vi "ActionVIOnSave.vi"(8 "error in (no error)":errorcluster, 11 "Device Item Ref in":T1 format="%.0x") -> (0 "error out":errorcluster, 3 "Device Item Ref out":T1 format="%.0x")   [LabVIEW 2016]
uses:
  <vilib>/NI Veristand/Custom Device API/Custom Device Item Ref.ctl
  UDP-Custom-Device System Explorer.lvlib
  <vilib>/NI VeriStand/Custom Device API/Custom Device API.lvlib
  Shared/Constants.vi
  Shared/UDP-Custom-Device Shared.lvlib
  <vilib>/NI VeriStand/Custom Device Tools/Custom Device Utility Library/Custom Device Utility Library.lvlib
  <vilib>/NI Veristand/Custom Device API/Get Item Property (Boolean).vi
  <vilib>/NI Veristand/Custom Device API/Get Item Property (Path).vi
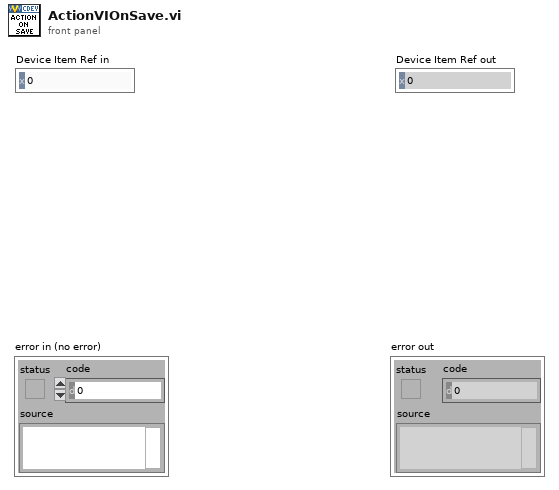
[diagram p1: front panel]
types:
  T1 = typedef "Custom Device API.lvlib/Custom Device Item Ref.ctl" = u64
  T2 = typedef "UDP-Custom-Device System Explorer.lvlib/XML - Header Data.ctl" = cluster{"Revision (\"Major.Minor.Fix.Build\")":string, "Creation Date (\"yyyy-mm-dd\")":string, "Controller Name":string}
  T3 = typedef "UDP-Custom-Device System Explorer.lvlib/XML - Group.ctl" = cluster{"Freq":i32, "Tx Channels":T4[], "Rx Channels":T4[]}
  T4 = typedef "UDP-Custom-Device System Explorer.lvlib/XML - Channel.ctl" = cluster{"Channel Name":string, "Data Type":u16, "Description":string, "Unit":string}
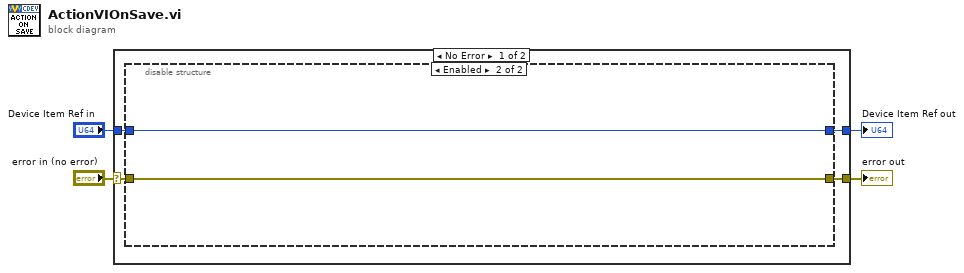
[diagram p0: block diagram]
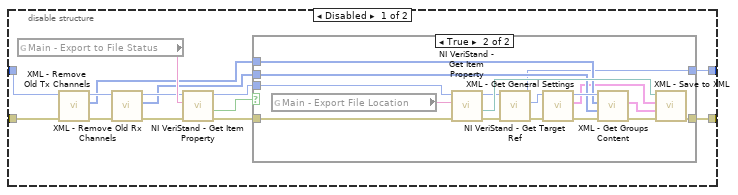
[diagram p2: hidden frame]
diagram:
  n1 = case shown="No Error" "error in (no error)" {
    selector: "error in (no error)" -> [w7 w45]
    tunnel: [w6 w45] -> w3
    tunnel: "Device Item Ref in" -> [w8 w44]
    tunnel: [w5 w44] -> w1
    frame No Error {
      n2 = disable-structure shown="Enabled" {
        disable-tunnel: w8 -> [w22 w43]
        disable-tunnel: w7 -> [w21 w42]
        disable-tunnel: [w10 w42] -> w6
        disable-tunnel: [w9 w43] -> w5
        frame Disabled {
          n3 = global read "Constants.vi" "Main - Export to File Status"() -> (w18:string)
          n4 = call "XML - Remove Old Tx Channels.vi"("error in (no error)"=w21, "Device Item Ref in"=w22) -> ("error out"=w20:errorcluster, "Tx Dependent Refs"=w12:T1[], "Device Item Ref out"=w19:T1)  [unwired: 7 in]
          n5 = call "XML - Remove Old Rx Channels.vi"("error in (no error)"=w20, "Device Item Ref in"=w19) -> ("error out"=w16:errorcluster, "Rx Dependent Refs"=w11:T1[], "Device Item Ref out"=w17:T1)  [unwired: 7 in]
          n6 = call-poly <vilib>:"NI VeriStand - Get Item Property.vi"("error in (no error)"=w16, "Property Name"=w18, "Item Ref in"=w17) -> ("error out"=w14:errorcluster, "Value"=w15:bool, "Item Ref out"=w13:T1)  [unwired: 5 in, 1 out]
          n7 = case shown="True" w15 {
            tunnel: w14 -> [w24 w41]
            tunnel: w13 -> [w23 w40]
            tunnel: w12 -> [_ w32]
            tunnel: w11 -> [_ w31]
            tunnel: [w24 w26] -> w10
            tunnel: [w23 w25] -> w9
            frame False {
            }
            frame True {
              n8 = global read "Constants.vi" "Main - Export File Location"() -> (w39:string)
              n9 = call-poly <vilib>:"NI VeriStand - Get Item Property.vi"("error in (no error)"=w41, "Property Name"=w39, "Item Ref in"=w40) -> ("error out"=w37:errorcluster, "Value"=w38:path, "Item Ref out"=w36:T1)  [unwired: 5 in, 1 out]
              n10 = call <vilib>:"NI VeriStand - Get Target Ref.vi"("error in"=w37, "Item Ref in"=w36) -> ("error out"=w34:errorcluster, "Target Ref"=w35:T1, "Item Ref out"=w25:T1)  [unwired: 6 in, 1 out]
              n11 = call "XML - Get General Settings.vi"("error in (no error)"=w34, "Target Ref in"=w35) -> ("error out"=w30:errorcluster, "XML Header Data"=w28:T2, "Target Ref out"=w33:T1)  [unwired: 7 in]
              n12 = call "XML - Get Groups Content.vi"("error in (no error)"=w30, "Rx"=w31, "Tx"=w32, "Target Ref In"=w33) -> ("error IO"=w29:errorcluster, "Groups"=w27:T3[])  [unwired: 5 in, 1 out]
              n13 = call "XML - Save to XML.vi"("error in"=w29, "Channel Groups"=w27, "XML Header Data"=w28, "XML File Path"=w38) -> ("error out"=w26:errorcluster)  [unwired: 7 in]
            }
          }
        }
        frame Enabled {
        }
      }
    }
    frame Error {
    }
  }
  "error out" <- w3
  "Device Item Ref out" <- w1
